vi "ISX3_Cmd_SetSetupSave.vi"(1 "Setup Slot":u8) -> (0 "set Setup Save Cmd":u8[](array[numeric]))   [LabVIEW 2012, in "Sciospec ISX3 Impedance Analyzer.lvlib"]
uses:
  Sciospec ISX3 Impedance Analyzer.lvlib
panel:
  # "This VI generates the command to save the configured setup to the device.\nThere are 255 available slots."
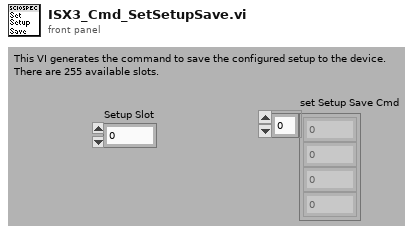
[diagram p1: front panel]
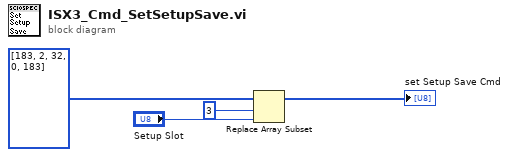
[diagram p0: block diagram]
diagram:
  n1 = Replace Array Subset(array=u8[] [183, 2, 32, 0, 183], new element="Setup Slot", index=3) -> (→"set Setup Save Cmd":u8[])
